vi "Deploy Stimulus Profile Session.vi"(8 "error in (no error)":errorcluster, 10 "Auto-Start (T)":bool=TRUE, 11 "Session Ref in":T1) -> (0 "error out":errorcluster, 2 "Deployed Session ID":string, 3 "Session Ref out":T1)   [LabVIEW 2020, in "NI_VS Sequence Execution Interface.lvlib"]
doc: "Deploys a stimulus profile session to an RT target."
uses:
  <vilib>/NI VeriStand/Execution/SequenceExecutionInterface/NI_VS Sequence Execution Interface.lvlib
  <vilib>/NI VeriStand/Execution/SequenceExecutionInterface/Stimulus Profile Session Ref.ctl
  NationalInstruments.VeriStand.ClientAPI
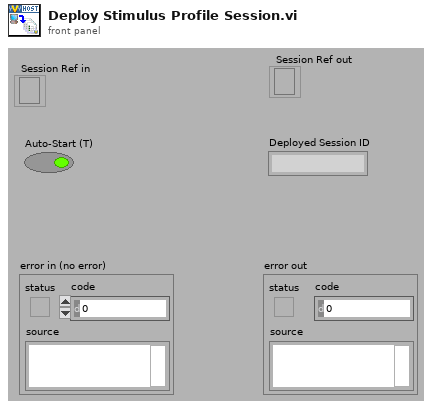
[diagram p1: front panel]
types:
  T1 = typedef "NI_VS Sequence Execution Interface.lvlib/Stimulus Profile Session Ref.ctl" = refnum<k24>
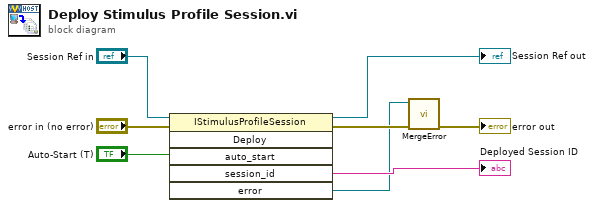
[diagram p0: block diagram]
diagram:
  n1 = invoke class="IStimulusProfileSession" method="Deploy"(reference="Session Ref in", error in="error in (no error)", "auto_start"="Auto-Start (T)") -> (reference out=→"Session Ref out":T1, error out=w8:errorcluster, "session_id"=→"Deployed Session ID":string, "error"=w2:refnum<k24>)  [unwired: 3 in, 2 out]
  n2 = call <vilib>:"MergeError.vi"("error in (no error)"=w8, "Error"=w2) -> ("error out"=→"error out":errorcluster)  [unwired: 9 out]
